vi "ManualControlL0SumnAdds.vi"() -> ()   [LabVIEW 2012]
uses:
  <vilib>/Utility/NIReport.llb/NI_report.lvclass
  <vilib>/Utility/NIReport.llb/HTML/NI_HTML.lvclass
  <instrlib>/Agilent 8000 Series/Public/Configure/Configure Math (Binary Operation).vi
  <instrlib>/Agilent 8000 Series/Agilent 8000 Series.lvlib
panel:
  in  "SET 2?":bool
  in  "SET?":bool
  in  "Clip_sel_b":u32=1
  in  "Ib_ClipVb":u32=63
  in  "Att gain":u32
  in  "Delay Enable":i32
  in  "Gen Active":bool=TRUE
  in  "Control\nGenNOsc":bool
  in  "Amp Scaler":dbl(slide)=1.3938122868656273 scale=0.1..250.0
  in  "Voltage Input":dbl(slide)=0.33316326530612245 scale=0.05..0.8
  in  "Enable 1":bool
  in  "Enable 0":bool
  in  "Enable 3":bool
  in  "Enable 2":bool
  in  "Enable 5":bool
  in  "Enable 4":bool
  in  "Enable 6":bool
  in  "stop":bool
  in  "Channels \nCombinations":i32[](array[numeric])=[3, 12, 48, 96, 7, 28, 112, 15, 120, 31, 124, 63, 126, 127]
  in  "index":i32
  out "element":i32
  in  "Instrument VISA in":T1={"AWG VISA"="AgilentGenerator1", "Oscilloscope  VISA "="AgilentOsciloscope", "Integration Board IP"="172.16.17.47", "connection ID"=refnum, "report out"=refnum, "report file path"=path "C:/Users/omartinez/Desktop/L0nL1_Results"}
  out "error out":errorcluster
  in  "error in (no error)":errorcluster
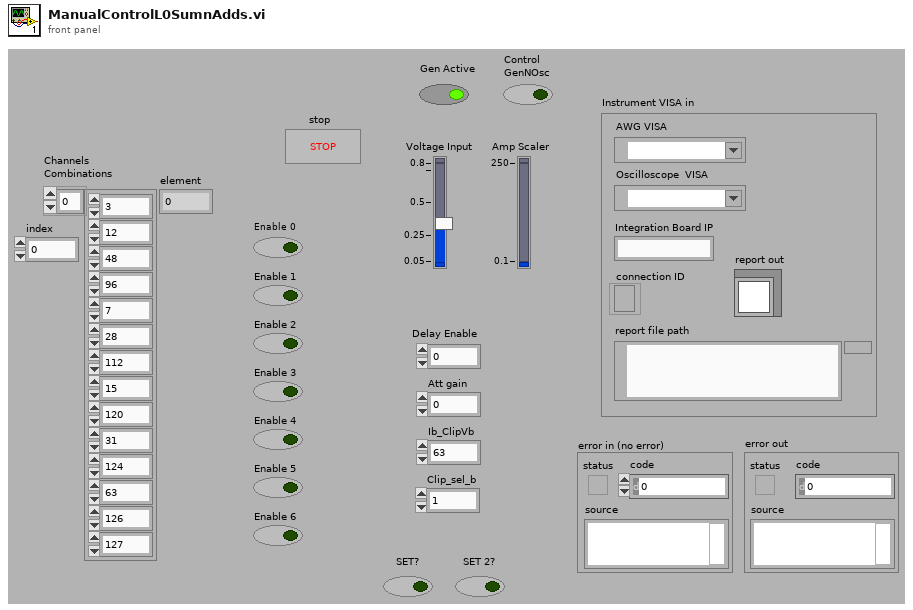
[diagram p1: front panel]
types:
  T1 = cluster{"AWG VISA":refnum<visa-resource-name>, "Oscilloscope  VISA ":refnum<visa-resource-name>, "Integration Board IP":string, "connection ID":refnum<k5>, "report out":refnum<class "NI_report.lvclass">, "report file path":path}
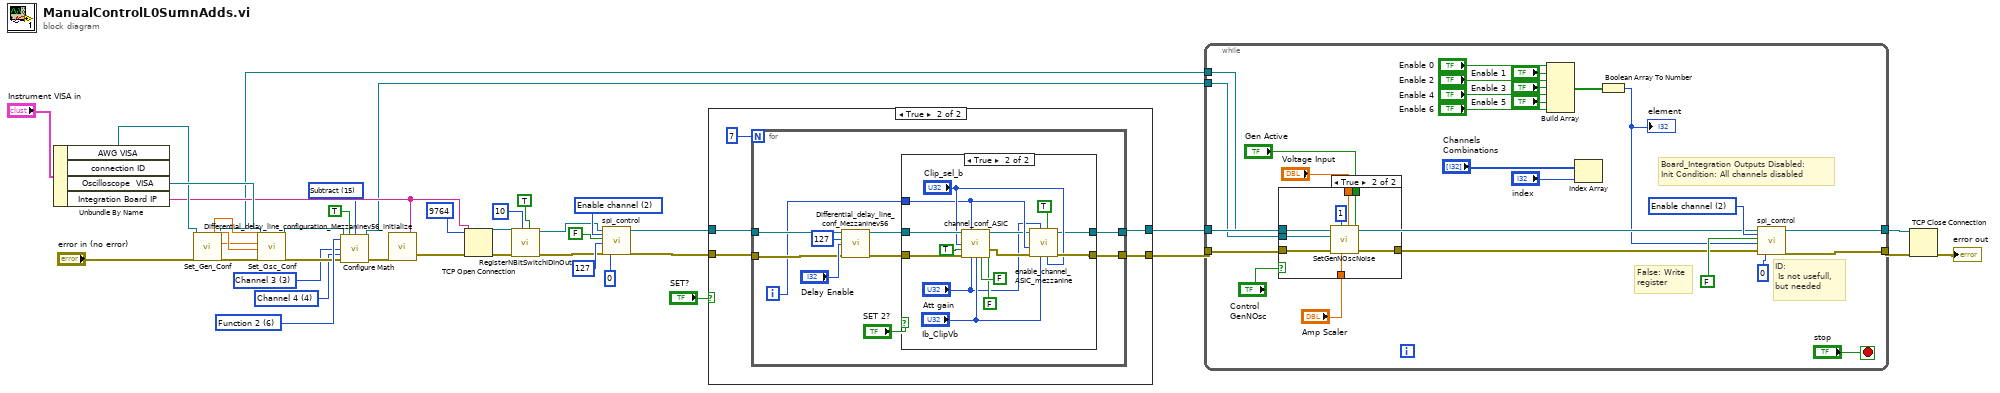
[diagram p0: block diagram]
diagram:
  w8 = u16 2 items=["Attenuation", "Clipping", "Enable channel", "Delay line", "ASIC"] ("Device")
  w21 = u16 6 items=["Function 1"=5, "Function 2"=6, "Function 3"=7, "Function 4"=8] ("Math Channel (5: Function 1)")
  w22 = u16 15 items=["Add"=12, "Divide"=13, "Multiply"=14, "Subtract"=15, "Common Mode"=16, "Versus"=17] ("Math Operation (12: Add)")
  w16 = 3 items=["Channel 1"=1, "Channel 2"=2, "Channel 3"=3, "Channel 4"=4] ("Channel (1: Channel 1)")
  w17 = 4 items=["Channel 1"=1, "Channel 2"=2, "Channel 3"=3, "Channel 4"=4] ("Channel (1: Channel 1)")
  n1 = Unbundle By Name("Instrument VISA in") -> ("AWG VISA"=w34:refnum<visa-resource-name>, "Oscilloscope  VISA"=w35:refnum<visa-resource-name>, "Integration Board IP"=w24:string)  [unwired: 1 out]
  n2 = call "Set_Gen_Conf.vi"("AWG VISA"=w34, "error in (no error)"="error in (no error)") -> ("Amplitude 1 OUT"=w32:dbl, "VISA resource name out"=w13:refnum<visa-resource-name>, "Pulse Width in seconds 1 OUT"=w31:dbl, "Trigger Level 1"=w30:dbl, "error out"=w37:errorcluster)  [unwired: 10 in, 3 out]
  n3 = call "Set_Osc_Conf.vi"("VISA resource name"=w35, "Amplitude IN"=w32, "Trigger Level IN"=w30, "Pulse Width in seconds IN"=w31, "error in (no error)"=w37) -> ("VISA resource name out"=w20:refnum<visa-resource-name>, "error out"=w19:errorcluster)  [unwired: 13 in]
  n4 = call-poly <instrlib>:"Configure Math.vi"("VISA resource name"=w20, "Enable Math Channel (T:Enable)"=TRUE, "Math Operation (12: Add)"=w22, "Math Channel (5: Function 1)"=w21, "Math Operand (1: Channel 1)"=w16, "Math Operand (2: Channel 2)"=w17, "error in (no error)"=w19) -> ("VISA resource name out"=w12:refnum<visa-resource-name>, "error out"=w18:errorcluster)  [unwired: 7 in]
  n5 = call "Differential_delay_line_configuration_Mezzaninev56_initialize.vi"("error in (no error)"=w18, "address"=w24) -> ("error out 2"=w29:errorcluster)
  n6 = TCP Open Connection(address=w24, remote port or service name=9764, error in (no error)=w29) -> (connection ID=w27:refnum<k5>, error out=w28:errorcluster)  [unwired: 2 in]
  n7 = call "RegisterNBitSwitchIDInOut.vi"("Switch Bit"=TRUE, "N Bit"=10, "error in (no error)"=w28, "connection ID"=w27) -> ("error out"=w5:errorcluster, "connection ID out"=w2:refnum<k5>)  [unwired: 5 in]
  n8 = call "spi_control.vi"("connection ID"=w2, "Device"=w8, "Read/#write"=FALSE, "Data"=127, "error in"=w5, "Id in"=0) -> ("connection ID out"=w3:refnum<k5>, "error out 2"=w4:errorcluster)  [unwired: 6 in, 6 out]
  n9 = case shown="True" "SET?" {
    tunnel: [w41 w45] -> w11
    tunnel: [w40 w44] -> w10
    tunnel: w4 -> [w41 w43]
    tunnel: w3 -> [w40 w42]
    frame False {
    }
    frame True {
      n10 = for {
        N: 7 -> [_]
        tunnel: w43 -> [w55]
        tunnel: w42 -> [w54]
        tunnel: [w51] -> w45
        tunnel: [w49] -> w44
        i -> [w50]
        n11 = call "Differential_delay_line_conf_Mezzaninev56.vi"("connection ID"=w54, "channel"=127, "Delay value"="Delay Enable", "error in (no error)"=w55) -> ("connection ID out"=w52:refnum<k5>, "error out 2"=w53:errorcluster)  [unwired: 4 in, 6 out]
        n12 = case shown="True" "SET 2?" {
          tunnel: w53 -> [w58 w72]
          tunnel: w52 -> [w57 w71]
          tunnel: [w58 w66] -> w51
          tunnel: w50 -> [_ w63]
          tunnel: [w57 w59] -> w49
          frame False {
          }
          frame True {
            n13 = call "channel_conf_ASIC.vi"("connection ID"=w71, "Ring"=w63, "Clip_sel_b"="Clip_sel_b", "CompBuf_en_b"=TRUE, "error out"=w72, "Att gain"="Att gain", "Ib_ClipVb"="Ib_ClipVb", "Clip_en_b"=FALSE, "Att_en_b"=FALSE) -> ("connection ID out"=w62:refnum<k5>, "error out 2"=w67:errorcluster)  [unwired: 2 in, 3 out]
            n14 = call "enable_channel_ASIC_mezzanine.vi"("Clip_sel_b"="Clip_sel_b", "maj/sum"=TRUE, "Ib_clipVb"="Ib_ClipVb", "Att gain"="Att gain", "error in"=w67, "Channel"=w63, "connection ID"=w62) -> ("error out"=w66:errorcluster, "connection ID out"=w59:refnum<k5>)  [unwired: 2 in, 1 out]
          }
        }
      }
    }
  }
  n15 = while {
    tunnel: w10 -> [w86]
    tunnel: w11 -> [w77]
    tunnel: [w84] -> w14
    tunnel: [w85] -> w15
    tunnel: w13 -> [w75]
    tunnel: w12 -> [w74]
    stop <- "stop" stop-if-true
    w97 = u16 2 items=["Attenuation", "Clipping", "Enable channel", "Delay line", "ASIC"] ("Device")
    # "False: Write\nregister"
    # "ID:\n Is not usefull, \nbut needed"
    # "Board_Integration Outputs Disabled:\nInit Condition: All channels disabled"
    n16 = case shown="True" "Control\nGenNOsc" {
      tunnel: w74 -> [_ w107]
      tunnel: w75 -> [_ w106]
      tunnel: w77 -> [w99 w105]
      tunnel: [w99 w104] -> w76
      tunnel: "Voltage Input" -> [_ w102]
      tunnel: "Amp Scaler" -> [_ w101]
      tunnel: "Gen Active" -> [_ w100]
      frame False {
      }
      frame True {
        n17 = call "SetGenNOscNoise.vi"("Enable Output"=w100, "Input Voltage"=w102, "Amp Scaler"=w101, "NChannels"=1, "error in (no error)"=w105, "Oscilloscope VISA"=w107, "Generator VISA"=w106) -> ("error out 2"=w104:errorcluster)  [unwired: 4 in]
      }
    }
    n18 = Build Array("Enable 0", "Enable 1", "Enable 2", "Enable 3", "Enable 4", "Enable 5", "Enable 6") -> (w95:bool[])
    n19 = Index Array(array="Channels \nCombinations", index="index") -> ()  [unwired: 1 out]
    n20 = Boolean Array To Number(Boolean array=w95) -> (number=w73:u32)
    "element" <- w73
    n21 = call "spi_control.vi"("connection ID"=w86, "Device"=w97, "Read/#write"=FALSE, "Data"=w73, "error in"=w76, "Id in"=0) -> ("connection ID out"=w85:refnum<k5>, "error out 2"=w84:errorcluster)  [unwired: 6 in, 6 out]
  }
  n22 = TCP Close Connection(connection ID=w15, error in (no error)=w14) -> (error out=→"error out":errorcluster)  [unwired: 1 in, 1 out]
